vi "burble.vi"() -> ()   [LabVIEW 2023]
panel:
  out "灯泡2":bool
  out "灯泡":bool
  in  "light switch":bool
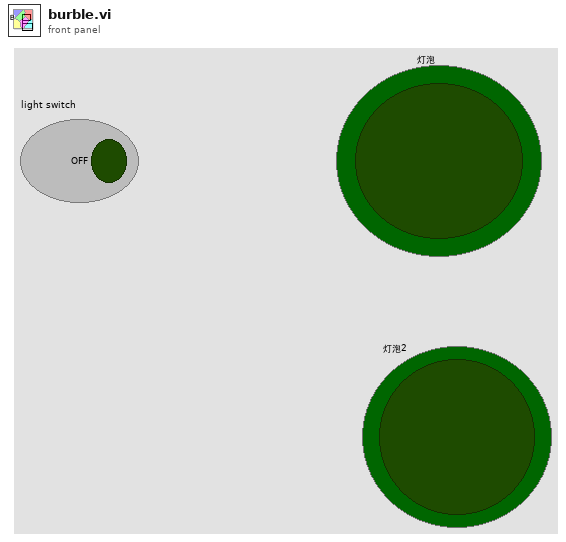
[diagram p1: front panel]
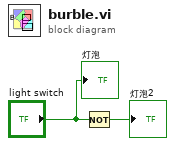
[diagram p0: block diagram]
diagram:
  n1 = Not(x="light switch") -> (.not. x?=→"灯泡2":bool)
  "灯泡" <- "light switch"
